vi "M Energy Storage.vi"(11 "NXT/EV3":T1) -> (3 "EV3 out":T1)   [LabVIEW 2016]
uses:
  <vilib>/NXT/Subs/LVHSConnector.ctl
  <vilib>/NXT/LegoClasses/BrickReference/BrickReference.lvclass
  <vilib>/NXT/Dual Mode Library/Waits/Wait_Num.vi
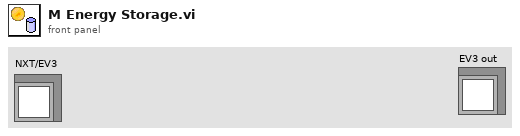
[diagram p1: front panel]
types:
  T1 = typedef "LVHSConnector.ctl" = refnum<class "BrickReference.lvclass">
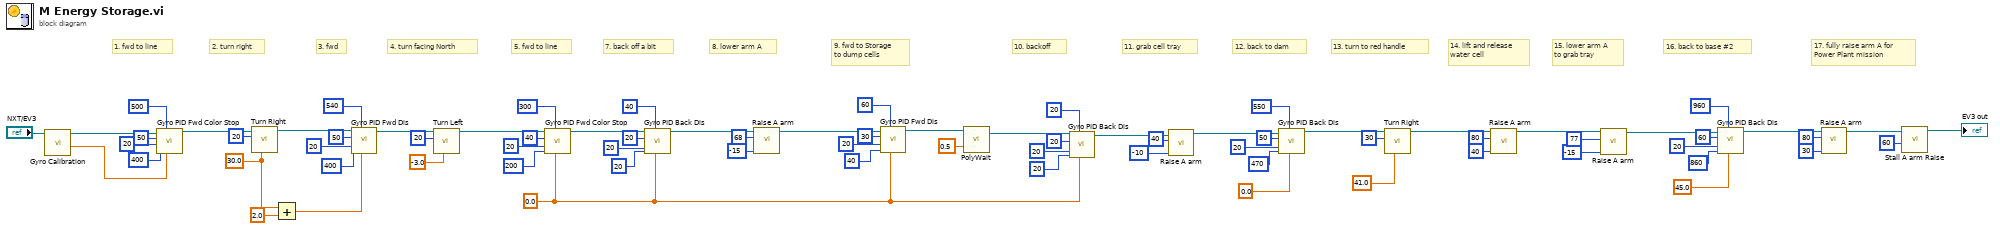
[diagram p0: block diagram]
diagram:
  w34 = sgl 0.0 ("Target angle")
  w37 = sgl 30.0 ("Turning angle")
  # "17. fully raise arm A for\nPower Plant mission"
  # "16. back to base #2"
  # "15. lower arm A\nto grab tray"
  # "14. lift and release\nwater cell"
  # "13. turn to red handle"
  # "12. back to dam"
  # "11. grab cell tray"
  # "10. backoff"
  # "9. fwd to Storage\nto dump cells"
  # "8. lower arm A"
  # "7. back off a bit"
  # "5. fwd to line"
  # "4. turn facing North"
  # "3. fwd"
  # "2. turn right"
  # "1. fwd to line"
  n1 = call "Gyro Calibration.vi"("NXT/EV3"="NXT/EV3") -> ("Degrees"=w72:sgl, "NXT/EV3"=w25:T1)  [unwired: 6 in, 1 out]
  n2 = call "Gyro PID Fwd Color Stop.vi"("Target angle"=w72, "Threshold to Color"=500, "Threshold to slow"=400, "Min. speed"=20, "Max. speed"=50, "EV3 in"=w25) -> ("EV3 out"=w71:T1)  [unwired: 5 in]
  n3 = call "Turn Right.vi"("Turning angle"=w37, "Motor B (right)"=i8 20, "EV3 in"=w71) -> ("EV3 out"=w69:T1)  [unwired: 8 in]
  n4 = Add(x=w37, y=sgl 2.0) -> (x+y=w35:sgl)
  n5 = call "Gyro PID Fwd Dis.vi"("Target angle"=w35, "Threshold to stop"=540, "Threshold to slow"=400, "Min. speed"=20, "Max. speed"=50, "EV3 in"=w69) -> ("EV3 out"=w64:T1)  [unwired: 5 in]
  n6 = call "Turn Left.vi"("Turning angle"=sgl -3.0, "Motor B (right)"=i8 20, "EV3 in"=w64) -> ("EV3 out"=w61:T1)  [unwired: 8 in]
  n7 = call "Gyro PID Fwd Color Stop.vi"("Target angle"=w34, "Threshold to Color"=300, "Threshold to slow"=200, "Min. speed"=20, "Max. speed"=40, "EV3 in"=w61) -> ("EV3 out"=w56:T1)  [unwired: 5 in]
  n8 = call "Gyro PID Back Dis.vi"("Target angle"=w34, "Threshold to stop"=40, "Threshold to slow"=20, "Min. speed"=20, "Max. speed"=20, "EV3 in"=w56) -> ("EV3 out"=w51:T1)  [unwired: 5 in]
  n9 = call "Raise A arm.vi"("Power"=i8 -15, "Rotation"=68, "EV3 in"=w51) -> ("EV3 out"=w23:T1)  [unwired: 8 in]
  n10 = call "Gyro PID Fwd Dis.vi"("Target angle"=w34, "Threshold to stop"=60, "Threshold to slow"=40, "Min. speed"=20, "Max. speed"=30, "EV3 in"=w23) -> ("EV3 out"=w44:T1)  [unwired: 5 in]
  n11 = call-poly <vilib>:"PolyWait.vi"("Time (1 sec)"=sgl 0.5, "NXT/EV3"=w44) -> ("NXT/EV3"=w42:T1)  [unwired: 2 in]
  n12 = call "Gyro PID Back Dis.vi"("Target angle"=w34, "Threshold to stop"=20, "Threshold to slow"=20, "Min. speed"=20, "Max. speed"=20, "EV3 in"=w42) -> ("EV3 out"=w32:T1)  [unwired: 5 in]
  n13 = call "Raise A arm.vi"("Power"=i8 -10, "Rotation"=40, "EV3 in"=w32) -> ("EV3 out"=w29:T1)  [unwired: 8 in]
  n14 = call "Gyro PID Back Dis.vi"("Target angle"=sgl 0.0, "Threshold to stop"=550, "Threshold to slow"=470, "Min. speed"=20, "Max. speed"=50, "EV3 in"=w29) -> ("EV3 out"=w17:T1)  [unwired: 5 in]
  n15 = call "Turn Right.vi"("Turning angle"=sgl 41.0, "Motor B (right)"=i8 30, "EV3 in"=w17) -> ("EV3 out"=w7:T1)  [unwired: 8 in]
  n16 = call "Raise A arm.vi"("Power"=i8 40, "Rotation"=80, "EV3 in"=w7) -> ("EV3 out"=w15:T1)  [unwired: 8 in]
  n17 = call "Raise A arm.vi"("Power"=i8 -15, "Rotation"=77, "EV3 in"=w15) -> ("EV3 out"=w9:T1)  [unwired: 8 in]
  n18 = call "Gyro PID Back Dis.vi"("Target angle"=sgl 45.0, "Threshold to stop"=960, "Threshold to slow"=860, "Min. speed"=20, "Max. speed"=60, "EV3 in"=w9) -> ("EV3 out"=w4:T1)  [unwired: 5 in]
  n19 = call "Raise A arm.vi"("Power"=i8 30, "Rotation"=80, "EV3 in"=w4) -> ("EV3 out"=w3:T1)  [unwired: 8 in]
  n20 = call "Stall A arm Raise.vi"("Power"=i8 60, "NXT/EV3"=w3) -> ("NXT/EV3"=→"EV3 out":T1)  [unwired: 9 in]
